vi "Pump Out Selection.vi"(6 "Module Type":enum16{"Feed Module", "Pump Module"}(ring), 8 "error in (no error)":errorcluster, 9 "Calibration":dbl, 10 "Speed":dbl, 11 "Pump Settings In":T1 {"Masterflex"."Pump Number" min=1.0 max=20.0 step=1.0; "Ismatech"."Pump Number" min=1.0 max=20.0 step=1.0; "ASIA Pump C"."channel" min=-1 max=1 step=1}) -> (0 "error out":errorcluster, 2 "Connection Error":bool, 3 "Pump Settings Out":T1 {"Masterflex"."Pump Number" min=1.0 max=20.0 step=1.0; "Ismatech"."Pump Number" min=1.0 max=20.0 step=1.0; "ASIA Pump C"."channel" min=-1 max=1 step=1})   [LabVIEW 2018, in "Pump Module.lvlib" / "Pump Module Engine.lvlib"]
uses:
  Pump Module Engine.lvlib
  Pump Settings Cluster.ctl
  Measure Instrument/PID 2 Output Enum.ctl
  Masterflex 7550-30/Controls/Settings Cluster.ctl
  Ismatec ISM 831C/Controls/Ismatech Settings Cluster.ctl
  VICI M50 Party Mode/Settings Cluster.ctl
  Tacmina QI/Tacmina QI DAQ Setting.ctl
  KNF Pump/Settings Cluster plus SIMDOS.ctl
  ASIA Pump/Pump Settings.ctl
  FLOM Pump/Settings Cluster.ctl
  SSI PR Class/SSI PR Settings Cluster.ctl
  Ismatec ISM 831C/Ismatec ISM 831C.lvlib
  Masterflex 7550-30/Masterflex 7550-30.lvlib
  VICI M50 Party Mode/VICI M6 M50 Party Mode.lvlib
  Tacmina QI/Tacmina QI.lvlib
  KNF Pump/KNF SIMDOS.lvlib
  ASIA Pump.lvlib
  FLOM Pump/FLOM Pump.lvlib
  SSI PR Class/SSI PR Pump.lvlib
  Pump Module.lvlib
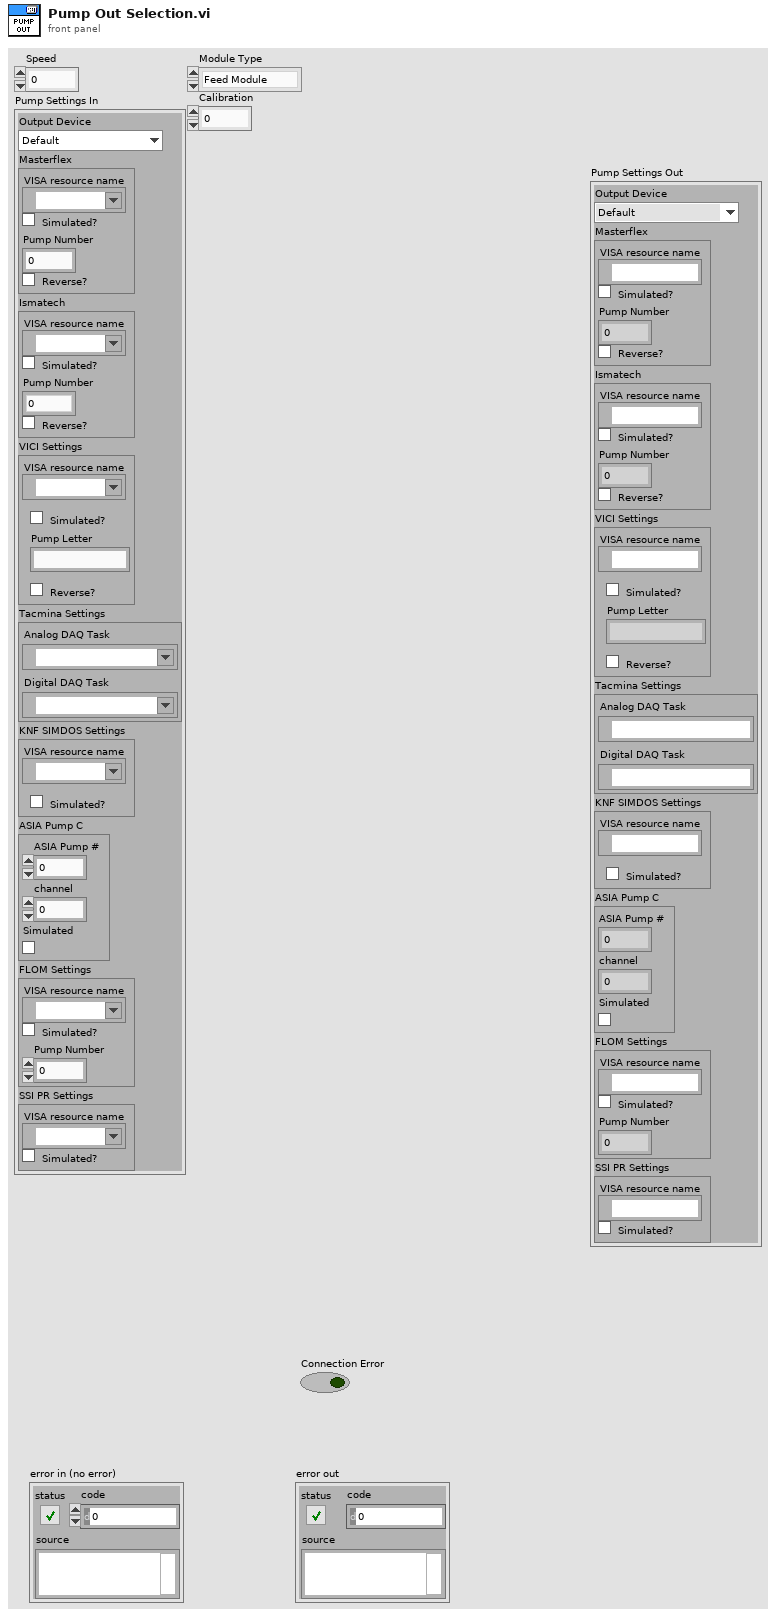
[diagram p1: front panel]
types:
  T1 = typedef "Pump Module.lvlib/Pump Settings Cluster.ctl" = cluster{"Output Device":T2, "Masterflex":T3, "Ismatech":T4, "VICI Settings":T5, "Tacmina Settings":T6, "KNF SIMDOS Settings":T7, "ASIA Pump C":T8, "FLOM Settings":T9, "SSI PR Settings":T10}
  T2 = typedef "PID 2 Output Enum.ctl" = enum16{"Default", "Ismatec ISM 831C", "Masterflex 7550-30", "VICI", "Tacmina QI", "KNF SIMDOS", "ASIA Type C", "FLOM UI-22-11", "SSI PR"}
  T3 = typedef "Masterflex 7550-30.lvlib/Settings Cluster.ctl" = cluster{"VISA resource name":refnum<visa-resource-name>, "Simulated?":bool, "Pump Number":dbl, "Reverse?":bool}
  T4 = typedef "Ismatec ISM 831C.lvlib/Ismatech Settings Cluster.ctl" = cluster{"VISA resource name":refnum<visa-resource-name>, "Simulated?":bool, "Pump Number":dbl, "Reverse?":bool}
  T5 = typedef "VICI M6 M50 Party Mode.lvlib/Settings Cluster.ctl" = cluster{"VISA resource name":refnum<visa-resource-name>, "Simulated?":bool, "Pump Letter":string, "Reverse?":bool}
  T6 = typedef "Tacmina QI.lvlib/Tacmina QI DAQ Setting.ctl" = cluster{"Analog DAQ Task":refnum<k21>, "Digital DAQ Task":refnum<k21>}
  T7 = typedef "KNF SIMDOS.lvlib/Settings Cluster plus SIMDOS.ctl" = cluster{"VISA resource name":refnum<visa-resource-name>, "Simulated?":bool}
  T8 = typedef "ASIA Pump.lvlib/Pump Settings.ctl" = cluster{"ASIA Pump #":i32, "channel":i32, "Simulated":bool}
  T9 = typedef "FLOM Pump.lvlib/Settings Cluster.ctl" = cluster{"VISA resource name":refnum<visa-resource-name>, "Simulated?":bool, "Pump Number":dbl}
  T10 = typedef "SSI PR Pump.lvlib/SSI PR Settings Cluster.ctl" = cluster{"VISA resource name":refnum<visa-resource-name>, "Simulated?":bool}
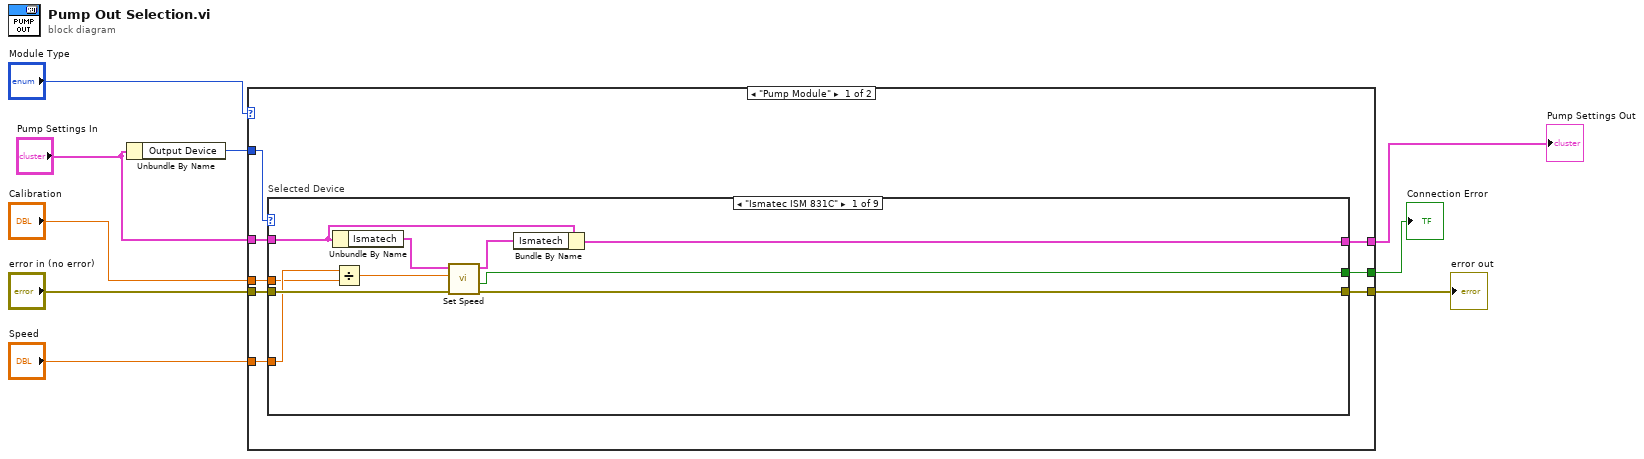
[diagram p0: block diagram]
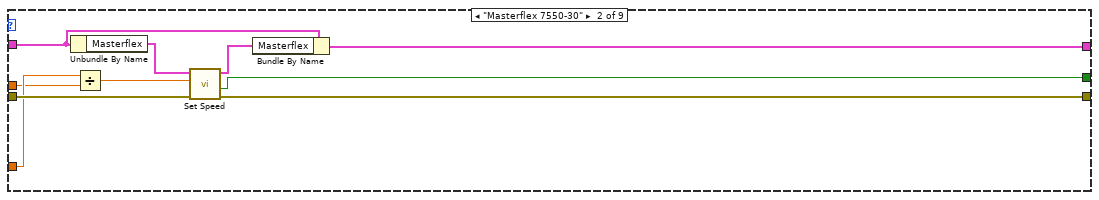
[diagram p2: hidden frame]
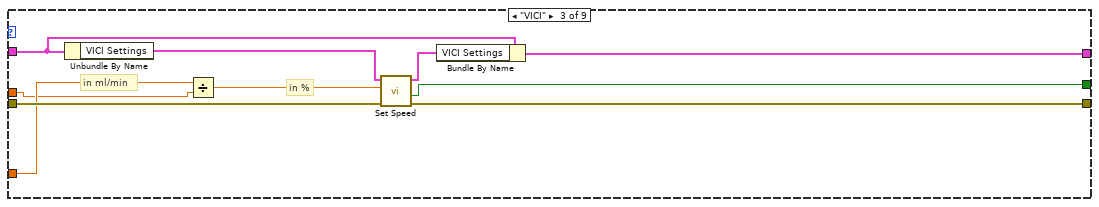
[diagram p3: hidden frame]
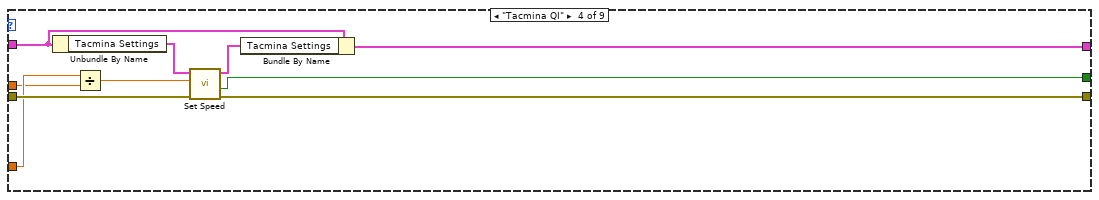
[diagram p4: hidden frame]
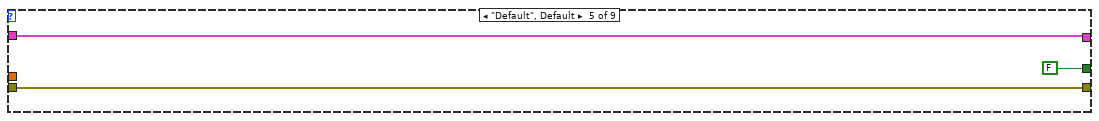
[diagram p5: hidden frame]
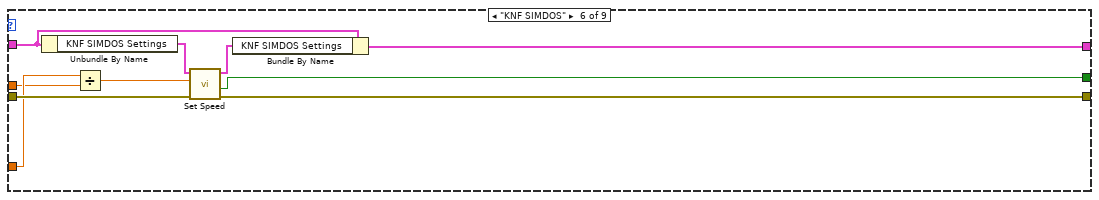
[diagram p6: hidden frame]
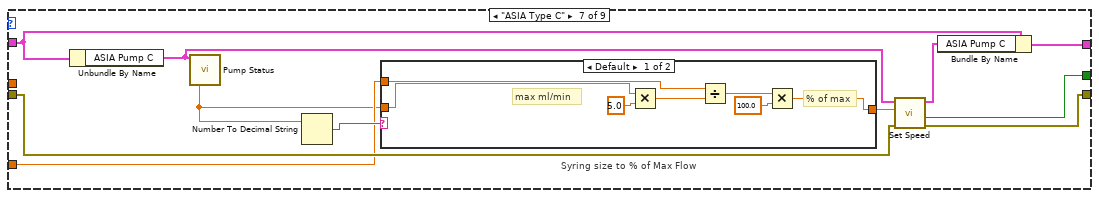
[diagram p7: hidden frame]
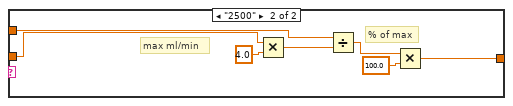
[diagram p8: hidden frame]
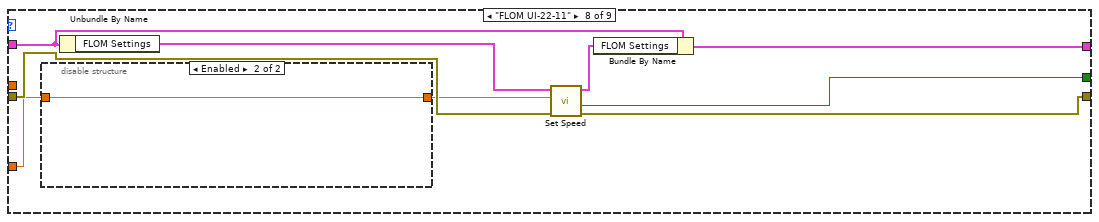
[diagram p9: hidden frame]
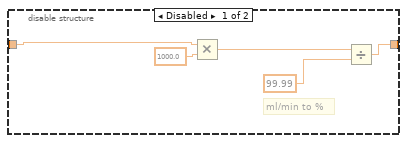
[diagram p10: hidden frame]
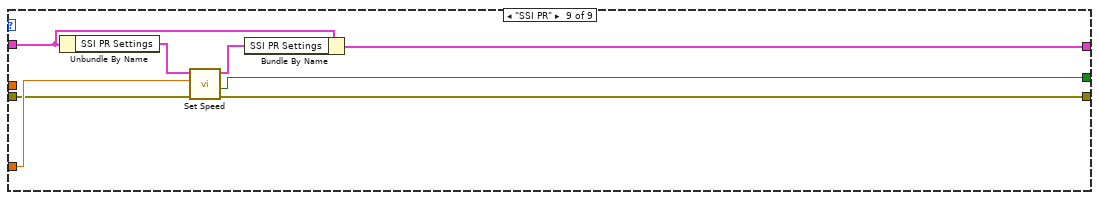
[diagram p11: hidden frame]
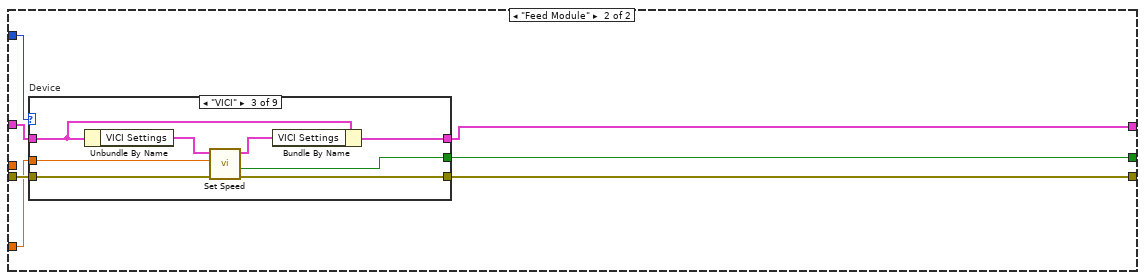
[diagram p12: hidden frame]
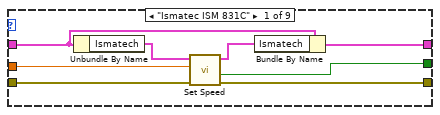
[diagram p13: hidden frame]
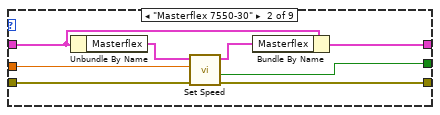
[diagram p14: hidden frame]
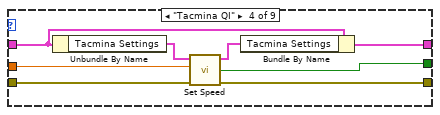
[diagram p15: hidden frame]
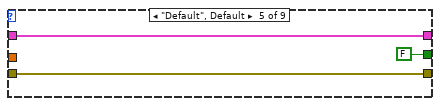
[diagram p16: hidden frame]
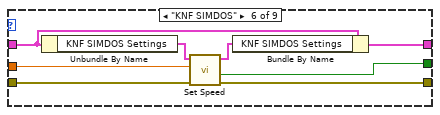
[diagram p17: hidden frame]
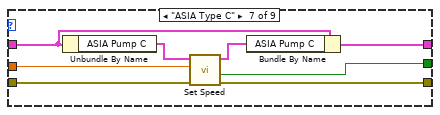
[diagram p18: hidden frame]
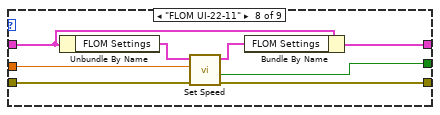
[diagram p19: hidden frame]
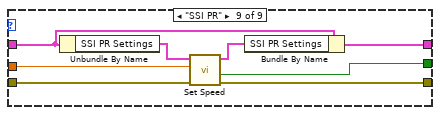
[diagram p20: hidden frame]
diagram:
  n1 = Unbundle By Name("Pump Settings In") -> ("Output Device"=w4:T2)
  n2 = case shown="\"Pump Module\"" "Module Type" {
    tunnel: [w17 w120] -> w9
    tunnel: [w16 w119] -> w8
    tunnel: "error in (no error)" -> [w15 w123]
    tunnel: "Pump Settings In" -> [w14 w124]
    tunnel: "Speed" -> [w13 w122]
    tunnel: [w12 w121] -> w2
    tunnel: w4 -> [w11 w125]
    tunnel: "Calibration" -> [w10 _]
    frame "Pump Module" {
      n3 = case "Selected Device" shown="\"Ismatec ISM 831C\"" w11 {
        tunnel: w13 -> [w20 w30 w39 w50 _ w63 w73 w96 w116]
        tunnel: w15 -> [w27 w33 w46 w56 w59 w69 w81 w102 w112]
        tunnel: [w26 w32 w45 w55 w59 w68 w80 w99 w113] -> w16
        tunnel: w14 -> [w25 w37 w42 w52 w60 w66 w76 w101 w118]
        tunnel: [w22 w36 w44 w54 w60 w65 w77 w98 w117] -> w12
        tunnel: [w21 w31 w41 w51 FALSE ("Connection Error") w64 w79 w100 w111] -> w17
        tunnel: w10 -> [w18 w28 w38 w48 _ w61 _ _ _]
        frame "Ismatec ISM 831C" {
          n4 = Unbundle By Name(w25) -> ("Ismatech"=w24:T4)
          n5 = Divide(x=w20, y=w18) -> (x/y=w19:dbl)
          n6 = call "Set Speed.vi"("error in (no error)"=w27, "Speed (%)"=w19, "Ismatech Settings"=w24) -> ("error out"=w26:errorcluster, "Connection Error"=w21:bool, "Ismatech Settings"=w23:T4)  [unwired: 6 in]
          n7 = Bundle By Name(cluster=w25, "Ismatech"=w23) -> (w22:T1)
        }
        frame "Masterflex 7550-30" {
          n8 = Unbundle By Name(w37) -> ("Masterflex"=w35:T3)
          n9 = Divide(x=w30, y=w28) -> (x/y=w29:dbl)
          n10 = call "Set Speed.vi"("error in (no error)"=w33, "speed"=w29, "Masterflex Settings in"=w35) -> ("error out"=w32:errorcluster, "Connection Error"=w31:bool, "Masterflex Settings out"=w34:T3)  [unwired: 6 in]
          n11 = Bundle By Name(cluster=w37, "Masterflex"=w34) -> (w36:T1)
        }
        frame "VICI" {
          # "in ml/min"
          # "in %"
          n12 = Unbundle By Name(w42) -> ("VICI Settings"=w47:T5)
          n13 = Divide(x=w39, y=w38) -> (x/y=w40:dbl)
          n14 = call "Set Speed.vi"("error in (no error)"=w46, "speed"=w40, "VICI Settings"=w47) -> ("error out"=w45:errorcluster, "Connection Error"=w41:bool, "VICI Settings"=w43:T5)  [unwired: 6 in]
          n15 = Bundle By Name(cluster=w42, "VICI Settings"=w43) -> (w44:T1)
        }
        frame "Tacmina QI" {
          n16 = Unbundle By Name(w52) -> ("Tacmina Settings"=w57:T6)
          n17 = Divide(x=w50, y=w48) -> (x/y=w49:dbl)
          n18 = call "Set Speed.vi"("error in"=w56, "Pump %"=w49, "Tacmina Settings in"=w57) -> ("error out"=w55:errorcluster, "Connection Error"=w51:bool, "Tacmina Settings out"=w53:T6)  [unwired: 6 in]
          n19 = Bundle By Name(cluster=w52, "Tacmina Settings"=w53) -> (w54:T1)
        }
        frame "Default", Default {
        }
        frame "KNF SIMDOS" {
          n20 = Unbundle By Name(w66) -> ("KNF SIMDOS Settings"=w70:T7)
          n21 = Divide(x=w63, y=w61) -> (x/y=w62:dbl)
          n22 = call "Set Speed.vi"("error in (no error)"=w69, "FlowRate"=w62, "KNF Settings"=w70) -> ("error out"=w68:errorcluster, "Connection Error"=w64:bool, "KNF Settings"=w67:T7)  [unwired: 6 in]
          n23 = Bundle By Name(cluster=w66, "KNF SIMDOS Settings"=w67) -> (w65:T1)
        }
        frame "ASIA Type C" {
          n24 = Unbundle By Name(w76) -> ("ASIA Pump C"=w72:T8)
          n25 = call "Pump Status.vi"("ASIA Pump C Settings in"=w72) -> ("syringeSize (ml)"=w71:sgl)  [unwired: 6 in, 8 out]
          n26 = Number To Decimal String(number=w71) -> (decimal integer string=w75:string)  [unwired: 1 in]
          n27 = case "Syring size to % of Max Flow" shown="Default" w75 {
            tunnel: w71 -> [w87 w91]
            tunnel: w73 -> [w86 w90]
            tunnel: [w82 w89] -> w74
            frame Default {
              # "% of max"
              # "max ml/min"
              n28 = Multiply(x=w87, y=5.0) -> (x*y=w85:dbl)
              n29 = Divide(x=w86, y=w85) -> (x/y=w84:dbl)
              n30 = Multiply(x=w84, y=100.0) -> (x*y=w82:dbl)
            }
            frame "2500" {
              # "% of max"
              # "max ml/min"
              n31 = Multiply(x=w91, y=4.0) -> (x*y=w94:dbl)
              n32 = Divide(x=w90, y=w94) -> (x/y=w93:dbl)
              n33 = Multiply(x=w93, y=100.0) -> (x*y=w89:dbl)
            }
          }
          n34 = call "Set Speed.vi"("error in (no error)"=w81, "Pump %"=w74, "ASIA Pump C Settings in"=w72) -> ("error out"=w80:errorcluster, "Connection Error"=w79:bool, "ASIA Pump C Settings out"=w78:T8)  [unwired: 6 in]
          n35 = Bundle By Name(cluster=w76, "ASIA Pump C"=w78) -> (w77:T1)
        }
        frame "FLOM UI-22-11" {
          n36 = disable-structure shown="Enabled" {
            disable-tunnel: [w108 w110] -> w97
            disable-tunnel: w96 -> [w106 w110]
            frame Disabled {
              # "ml/min to %"
              n37 = Multiply(x=w106, y=1000.0) -> (x*y=w105:dbl)
              n38 = Divide(x=w105, y=99.99) -> (x/y=w108:dbl)
            }
            frame Enabled {
            }
          }
          n39 = Unbundle By Name(w101) -> ("FLOM Settings"=w103:T9)
          n40 = call "Set Speed.vi"("error in (no error)"=w102, "speed"=w97, "FLOM Settings in"=w103) -> ("error out"=w99:errorcluster, "Connection Error"=w100:bool, "FLOM Settings out"=w104:T9)  [unwired: 6 in]
          n41 = Bundle By Name(cluster=w101, "FLOM Settings"=w104) -> (w98:T1)
        }
        frame "SSI PR" {
          n42 = Unbundle By Name(w118) -> ("SSI PR Settings"=w115:T10)
          n43 = call "Set Speed.vi"("error in (no error)"=w112, "speed (ml/min)"=w116, "SSI PR Settings"=w115) -> ("error out"=w113:errorcluster, "Connection Error"=w111:bool, "SSI PR Settings"=w114:T10)  [unwired: 6 in]
          n44 = Bundle By Name(cluster=w118, "SSI PR Settings"=w114) -> (w117:T1)
        }
      }
    }
    frame "Feed Module" {
      n45 = case "Device" shown="\"VICI\"" w125 {
        tunnel: w122 -> [w127 w135 w148 w156 _ w168 w176 w180 w186]
        tunnel: w123 -> [w133 w137 w147 w155 w159 w166 w171 w181 w190]
        tunnel: [w132 w136 w146 w154 w159 w163 w173 w177 w189] -> w119
        tunnel: w124 -> [w131 w141 w143 w151 w160 w165 w175 w182 w192]
        tunnel: [w128 w140 w145 w153 w160 w161 w174 w179 w191] -> w121
        tunnel: [w126 w134 w142 w150 FALSE ("Connection Error") w162 w172 w178 w185] -> w120
        frame "Ismatec ISM 831C" {
          n46 = Unbundle By Name(w131) -> ("Ismatech"=w130:T4)
          n47 = call "Set Speed.vi"("error in (no error)"=w133, "Speed (%)"=w127, "Ismatech Settings"=w130) -> ("error out"=w132:errorcluster, "Connection Error"=w126:bool, "Ismatech Settings"=w129:T4)  [unwired: 6 in]
          n48 = Bundle By Name(cluster=w131, "Ismatech"=w129) -> (w128:T1)
        }
        frame "Masterflex 7550-30" {
          n49 = Unbundle By Name(w141) -> ("Masterflex"=w139:T3)
          n50 = call "Set Speed.vi"("error in (no error)"=w137, "speed"=w135, "Masterflex Settings in"=w139) -> ("error out"=w136:errorcluster, "Connection Error"=w134:bool, "Masterflex Settings out"=w138:T3)  [unwired: 6 in]
          n51 = Bundle By Name(cluster=w141, "Masterflex"=w138) -> (w140:T1)
        }
        frame "VICI" {
          n52 = Unbundle By Name(w143) -> ("VICI Settings"=w149:T5)
          n53 = call "Set Speed.vi"("error in (no error)"=w147, "speed"=w148, "VICI Settings"=w149) -> ("error out"=w146:errorcluster, "Connection Error"=w142:bool, "VICI Settings"=w144:T5)  [unwired: 6 in]
          n54 = Bundle By Name(cluster=w143, "VICI Settings"=w144) -> (w145:T1)
        }
        frame "Tacmina QI" {
          n55 = Unbundle By Name(w151) -> ("Tacmina Settings"=w157:T6)
          n56 = call "Set Speed.vi"("error in"=w155, "Pump %"=w156, "Tacmina Settings in"=w157) -> ("error out"=w154:errorcluster, "Connection Error"=w150:bool, "Tacmina Settings out"=w152:T6)  [unwired: 6 in]
          n57 = Bundle By Name(cluster=w151, "Tacmina Settings"=w152) -> (w153:T1)
        }
        frame "Default", Default {
        }
        frame "KNF SIMDOS" {
          n58 = Unbundle By Name(w165) -> ("KNF SIMDOS Settings"=w167:T7)
          n59 = call "Set Speed.vi"("error in (no error)"=w166, "FlowRate"=w168, "KNF Settings"=w167) -> ("error out"=w163:errorcluster, "Connection Error"=w162:bool, "KNF Settings"=w164:T7)  [unwired: 6 in]
          n60 = Bundle By Name(cluster=w165, "KNF SIMDOS Settings"=w164) -> (w161:T1)
        }
        frame "ASIA Type C" {
          n61 = Unbundle By Name(w175) -> ("ASIA Pump C"=w170:T8)
          n62 = call "Set Speed.vi"("error in (no error)"=w171, "Pump %"=w176, "ASIA Pump C Settings in"=w170) -> ("error out"=w173:errorcluster, "Connection Error"=w172:bool, "ASIA Pump C Settings out"=w169:T8)  [unwired: 6 in]
          n63 = Bundle By Name(cluster=w175, "ASIA Pump C"=w169) -> (w174:T1)
        }
        frame "FLOM UI-22-11" {
          n64 = Unbundle By Name(w182) -> ("FLOM Settings"=w184:T9)
          n65 = call "Set Speed.vi"("error in (no error)"=w181, "speed"=w180, "FLOM Settings in"=w184) -> ("error out"=w177:errorcluster, "Connection Error"=w178:bool, "FLOM Settings out"=w183:T9)  [unwired: 6 in]
          n66 = Bundle By Name(cluster=w182, "FLOM Settings"=w183) -> (w179:T1)
        }
        frame "SSI PR" {
          n67 = Unbundle By Name(w192) -> ("SSI PR Settings"=w187:T10)
          n68 = call "Set Speed.vi"("error in (no error)"=w190, "speed (ml/min)"=w186, "SSI PR Settings"=w187) -> ("error out"=w189:errorcluster, "Connection Error"=w185:bool, "SSI PR Settings"=w188:T10)  [unwired: 6 in]
          n69 = Bundle By Name(cluster=w192, "SSI PR Settings"=w188) -> (w191:T1)
        }
      }
    }
  }
  "Connection Error" <- w9
  "error out" <- w8
  "Pump Settings Out" <- w2
